vi "progress string(SubVI).vi"(10 "String 3":string, 11 "String in":string) -> (3 "String out":string)   [LabVIEW 2018, in "Application.lvlib"]
uses:
  Application.lvlib
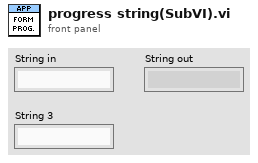
[diagram p1: front panel]
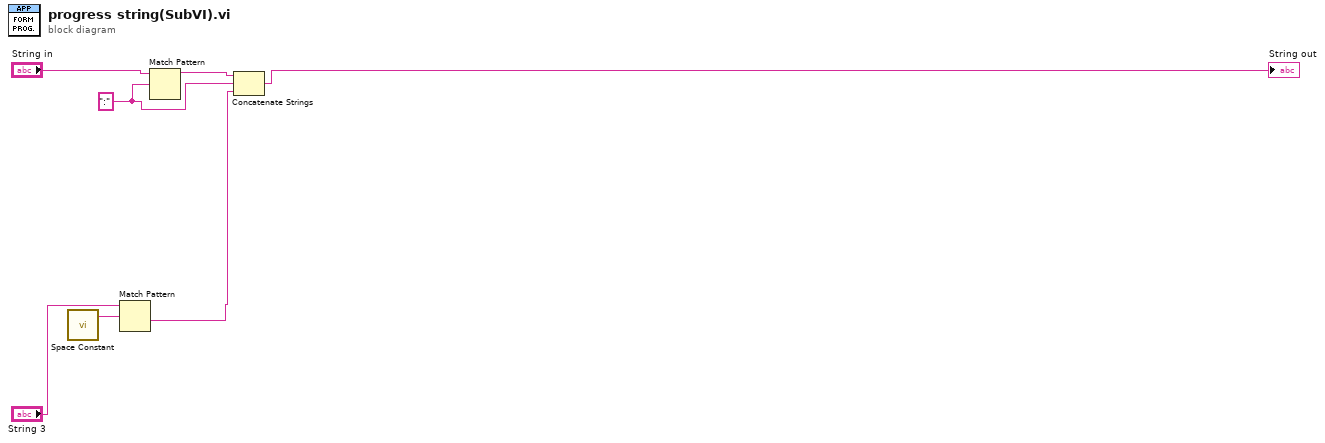
[diagram p0: block diagram]
diagram:
  w7 = ":" ("regular expression")
  n1 = call <vilib>:"Space Constant.vi"() -> ("String"=w2:string)
  n2 = Match Pattern(string="String 3", regular expression=w2) -> (after substring=w6:string)  [unwired: 1 in, 3 out]
  n3 = Match Pattern(string="String in", regular expression=w7) -> (before substring=w3:string)  [unwired: 1 in, 3 out]
  n4 = Concatenate Strings(w3, w7, w6) -> (→"String out":string)
